vi "Get Pin Status_UI Actor.vi"(8 "error in (no error)":errorcluster, 11 "UI Actor in":refnum<class "UI Actor.lvclass">) -> (0 "error out":errorcluster, 3 "UI Actor out":refnum<class "UI Actor.lvclass">)   [LabVIEW 2020, in "UI Actor.lvlib" / "UI Actor.lvclass"]
uses:
  UI Actor.lvclass
  UI Actor.lvclass/UI Actor.ctl
  Abstract/Serial Device/Serial Device.lvclass
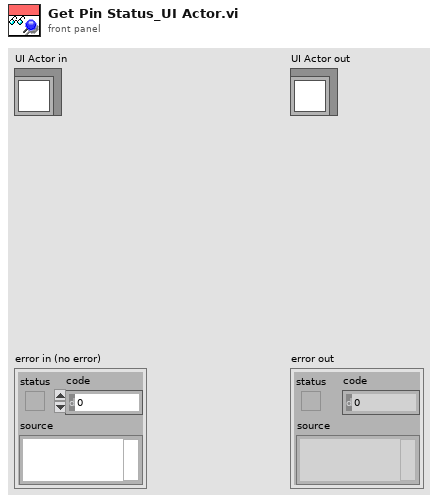
[diagram p1: front panel]
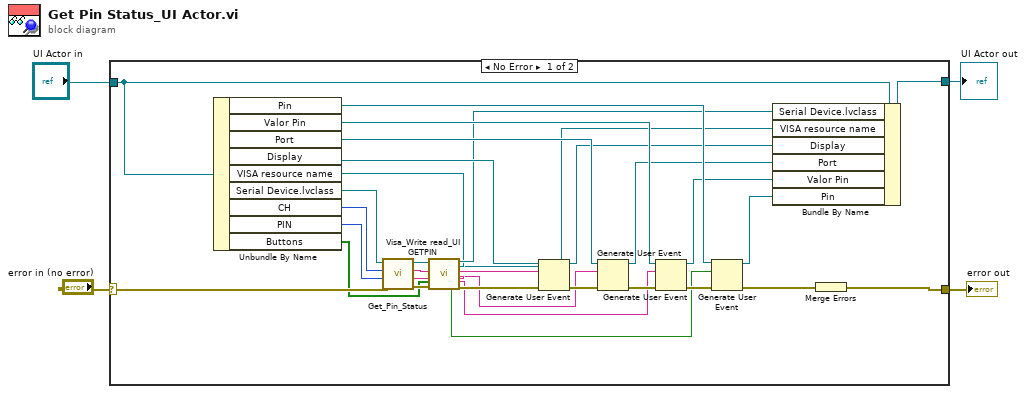
[diagram p0: block diagram]
diagram:
  n1 = case shown="No Error" "error in (no error)" {
    selector: "error in (no error)" -> [w30 w38]
    tunnel: [w32 w38] -> w3
    tunnel: [w36 w37] -> w1
    tunnel: "UI Actor in" -> [w31 w37]
    frame No Error {
      n2 = Unbundle By Name(w31) -> ("Pin"=w23:refnum<user-event>, "Valor Pin"=w22:refnum<user-event>, "Port"=w27:refnum<user-event>, "Display"=w34:refnum<user-event>, "VISA resource name"=w13:refnum<visa-resource-name>, "Serial Device.lvclass"=w35:refnum<class "Serial Device.lvclass">, "CH"=w25:i32, "PIN"=w26:i32, "Buttons"=w5:bool[])
      n3 = call-dynamic "Get_Pin_Status.vi"("error in (no error)"=w30, "PIN"=w26, "CH"=w25, "Serial Device in"=w35) -> ("error out"=w15:errorcluster, "Expected Response"=w10:string, "Command to Send"=w11:string, "Serial Device out"=w17:refnum<class "Serial Device.lvclass">)  [unwired: 4 in]
      n4 = call-dynamic "Visa_Write read_UI GETPIN.vi"("Serial Device in"=w17, "VISA resource name"=w13, "Command to Send"=w11, "Expected Response"=w10, "Buttons"=w5, "error in (no error)"=w15) -> ("Valor pin"=w6:bool, "Serial Device out"=w16:refnum<class "Serial Device.lvclass">, "VISA resource name"=w12:refnum<visa-resource-name>, "Response"=w9:string, "Port"=w8:string, "PIN"=w7:string, "error out"=w14:errorcluster)  [unwired: 7 in]
      n5 = Generate User Event(user event=w34, event data cluster=w9, error in=w14) -> (user event out=w18:refnum<user-event>, error out=w33:errorcluster)  [unwired: 1 in]
      n6 = Generate User Event(user event=w27, event data cluster=w8, error in=w33) -> (user event out=w19:refnum<user-event>, error out=w29:errorcluster)  [unwired: 1 in]
      n7 = Generate User Event(user event=w22, event data cluster=w7, error in=w29) -> (user event out=w20:refnum<user-event>, error out=w28:errorcluster)  [unwired: 1 in]
      n8 = Generate User Event(user event=w23, event data cluster=w6, error in=w28) -> (user event out=w21:refnum<user-event>, error out=w24:errorcluster)  [unwired: 1 in]
      n9 = Bundle By Name(cluster=w31, "Serial Device.lvclass"=w16, "VISA resource name"=w12, "Display"=w18, "Port"=w19, "Valor Pin"=w20, "Pin"=w21) -> (w36:refnum<class "UI Actor.lvclass">)
      n10 = Merge Errors(w24) -> (w32:errorcluster)
    }
    frame Error {
    }
  }
  "error out" <- w3
  "UI Actor out" <- w1
